vi "selectangle.vi"(0 "X Robot":dbl, 1 "Y Robot":dbl, 2 "Robot Heading (Degrees)":dbl, 3 "X Waypoint":dbl, 4 "Y Waypoint":dbl) -> (5 "Target Heading":dbl)   [LabVIEW 2010]
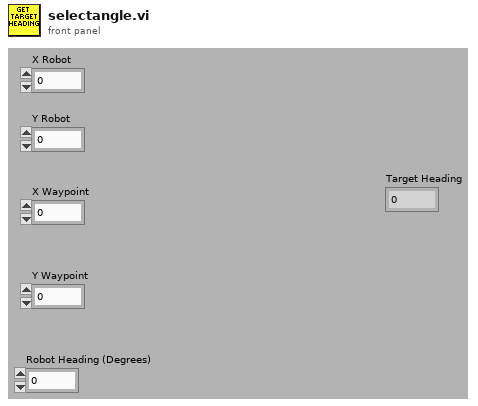
[diagram p1: front panel]
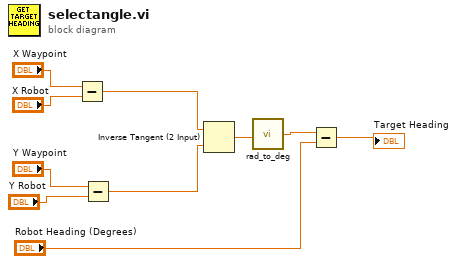
[diagram p0: block diagram]
diagram:
  n1 = Subtract(x="X Waypoint", y="X Robot") -> (x-y=w10:dbl)
  n2 = Subtract(x="Y Waypoint", y="Y Robot") -> (x-y=w9:dbl)
  n3 = Inverse Tangent (2 Input)(1:w9, 2:w10) -> (0:w7:dbl)
  n4 = call "rad_to_deg.vi"("Radians"=w7) -> ("Degrees"=w2:dbl)
  n5 = Subtract(x=w2, y="Robot Heading (Degrees)") -> (x-y=→"Target Heading":dbl)
